vi "Child_CreateReference.vi"(0 "ObjectReferenceToTest(Ignored If Empty)":variant, 5 "CreateMethod":T1(ring), 7 "Object name":string, 11 "error in (no error)":errorcluster) -> (4 "ObjectReferenceAsVariant":variant, 6 "NewObjectCreated":bool, 15 "error out":errorcluster)   [LabVIEW 2019, in "Child.lvclass"]
doc: "This VI is used by the Debug Spawning VI, to create a DVR reference for this objects attributes."
uses:
  Child.lvclass
  Child.lvclass/Child.ctl
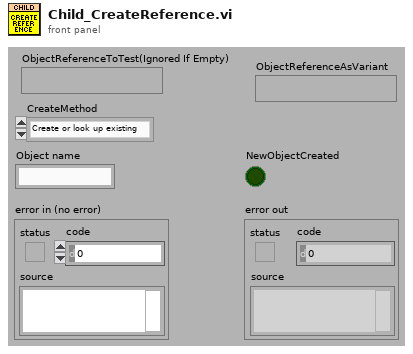
[diagram p1: front panel]
types:
  T1 = enum16{"Create or look up existing", "Look up existing"}
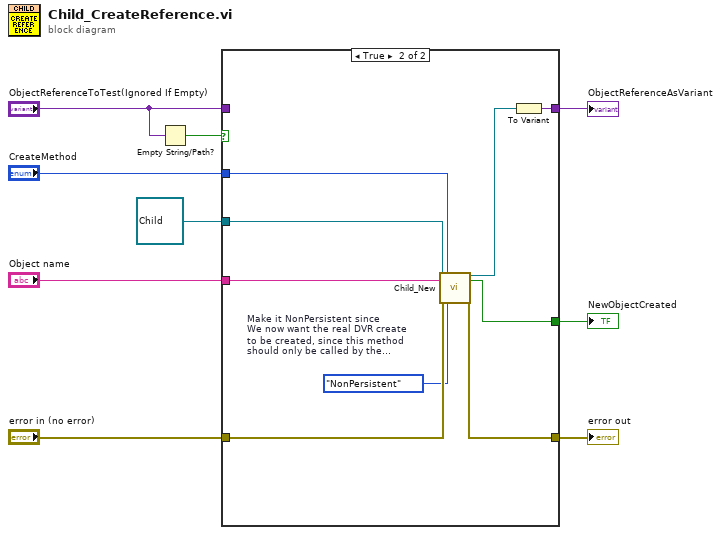
[diagram p0: block diagram]
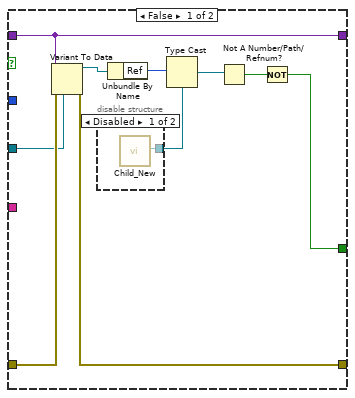
[diagram p2: hidden frame]
diagram:
  n1 = Empty String/Path?(string/path="ObjectReferenceToTest(Ignored If Empty)") -> (empty?=w3:bool)
  n2 = case shown="True" w3 {
    tunnel: "CreateMethod" -> [_ w29]
    tunnel: "error in (no error)" -> [w18 w28]
    tunnel: [w17 w27] -> w7
    tunnel: "Object name" -> [_ w26]
    tunnel: [w13 w25] -> w5
    tunnel: [w16 w23] -> w4
    tunnel: "ObjectReferenceToTest(Ignored If Empty)" -> [w16 _]
    tunnel: refnum<class "Child.lvclass"> refnum ("reference in") -> [w15 w21]
    frame False {
      n3 = Variant To Data(error in=w18, type=w15, Variant=w16) -> (data=w12:refnum<class "Child.lvclass">, error out=w17:errorcluster)
      n4 = disable-structure shown="Disabled" {
        disable-tunnel: [w20 _] -> w10
        frame Disabled {
          n5 = call "Child_New.vi"() -> ("DVRRefOut"=w20:refnum<data-value>)  [unwired: 16 in, 3 out]
        }
        frame Enabled {
        }
      }
      n6 = Unbundle By Name(w12) -> ("Ref"=w11:u32)
      n7 = Type Cast(type=w10, x=w11) -> (*(type *) &x=w19:refnum<data-value>)
      n8 = Not A Number/Path/Refnum?(number/path/refnum=w19) -> (NaN/Path/Refnum?=w14:bool)
      n9 = Not(x=w14) -> (.not. x?=w13:bool)
    }
    frame True {
      w22 = enum16{"Default", "Persistent", "NonPersistent"}."NonPersistent"  # Make it NonPersistent since We now want the real DVR create to be created, since this method should only be called by the persistent process
      n10 = call "Child_New.vi"("reference in"=w21, "Object name"=w26, "error in (no error)"=w28, "CreateMethod(Create or look up existing)"=w29, "Persistent/Debugging(Default)"=w22) -> ("reference out"=w24:refnum<class "Child.lvclass">, "NewObjectCreated"=w25:bool, "error out"=w27:errorcluster)  [unwired: 11 in, 1 out]
      n11 = To Variant(anything=w24) -> (Variant=w23:variant)
    }
  }
  "error out" <- w7
  "NewObjectCreated" <- w5
  "ObjectReferenceAsVariant" <- w4
